vi "Initialize Hardware References.vi"(8 "error in (no error)":errorcluster, 11 "Hardware Resources In":T1={"Piezo Serial Number"=41848555, "MG17Piezo"=refnum, "Setpoint (um)"=0.0}) -> (0 "error out":errorcluster, 3 "Hardware Resources Out":T1={"Piezo Serial Number"=41848555, "MG17Piezo"=refnum, "Setpoint (um)"=0.0})   [LabVIEW 2013, in "Piezo.lvlib"]
uses:
  Piezo.lvlib
  Hardware Configuration.ctl
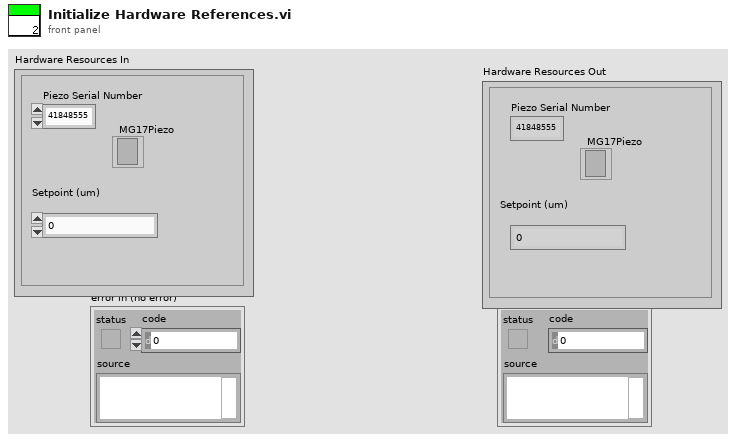
[diagram p1: front panel]
types:
  T1 = typedef "Piezo.lvlib/Hardware Configuration.ctl" = cluster{"Piezo Serial Number":i32, "MG17Piezo":refnum<k7>, "Setpoint (um)":sgl}
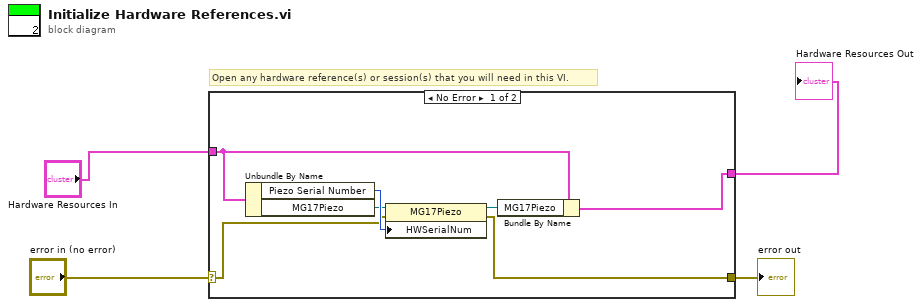
[diagram p0: block diagram]
diagram:
  # "Open any hardware reference(s) or session(s) that you will need in this VI."
  n1 = case shown="No Error" "error in (no error)" {
    selector: "error in (no error)" -> [w6 w13]
    tunnel: [w5 w13] -> w3
    tunnel: "Hardware Resources In" -> [w9 w12]
    tunnel: [w7 w12] -> w1
    frame No Error {
      n2 = Unbundle By Name(w9) -> ("Piezo Serial Number"=w11:i32, "MG17Piezo"=w10:refnum<k7>)
      n3 = property class="MG17Piezo"(reference=w10, error in=w6, "HWSerialNum"=w11) -> (reference out=w8:refnum<k7>, error out=w5:errorcluster)
      n4 = Bundle By Name(cluster=w9, "MG17Piezo"=w8) -> (w7:T1)
    }
    frame Error {
    }
  }
  "error out" <- w3
  "Hardware Resources Out" <- w1
